vi "Cross_Moments_for_slip.vi"(0 "U":dbl[](array[numeric]) format="%.2f", 1 "W":dbl[](array[numeric]) format="%.2f", 2 "Block No":i32=1, 5 "Shift in":dbl[](array[numeric]) format="%.2f") -> (14 "Correlations Only":string[](array[string]), 19 "Shift out":dbl[](array[numeric]) format="%.2f")   [LabVIEW 2010]
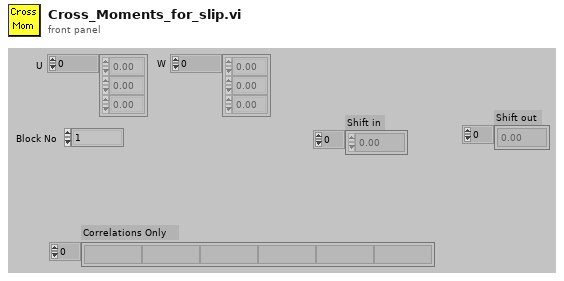
[diagram p1: front panel]
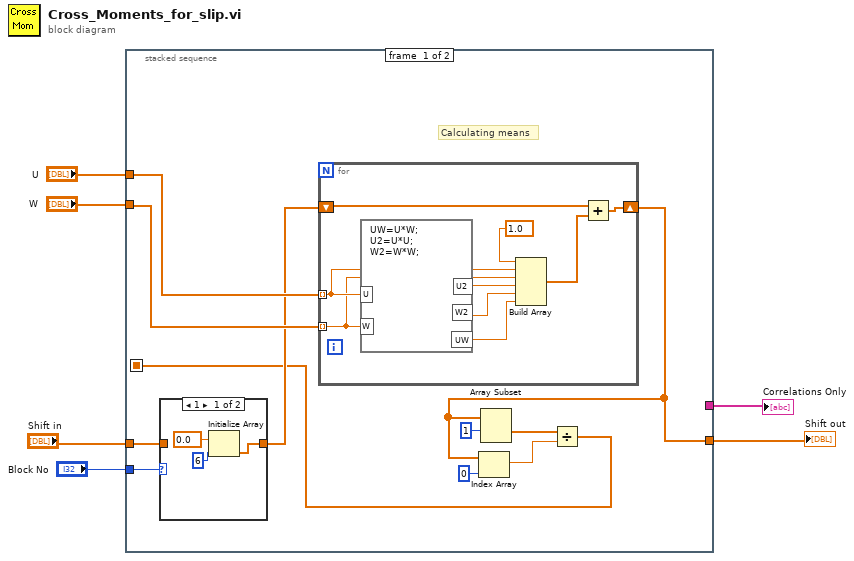
[diagram p0: block diagram]
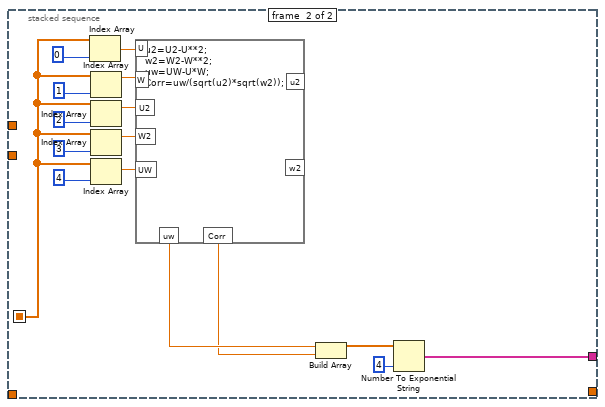
[diagram p3: hidden frame]
diagram:
  n1 = stacked-sequence {
    seq-local: [w7 _] -> [_ w41]
    tunnel: "U" -> [w17 _]
    tunnel: [w10 _] -> w5
    tunnel: "Shift in" -> [w13 _]
    tunnel: "W" -> [w16 _]
    tunnel: "Block No" -> [w15 _]
    tunnel: [_ w31] -> w1
    frame #0 {
      # "Calculating means"
      n2 = case shown="1" w15 {
        tunnel: [w18 w21] -> w14
        tunnel: w13 -> [_ w21]
        frame 1 {
          n3 = Initialize Array(0.0 ("Element Data"), 6 ("Dimension Size")) -> (w18:dbl[])
        }
        frame 2, Default {
        }
      }
      n4 = for {
        shift-right: [w26] -> w10
        shift-left: w14 -> [w25]
        tunnel: w17 -> [w24] mode=indexing
        tunnel: w16 -> [w23] mode=indexing
        n5 = formula code="UW=U*W;\nU2=U*U;\nW2=W*W;"("W"=w23, "U"=w24) -> ("UW"=w28:dbl, "U2"=w30:dbl, "W2"=w29:dbl)
        n6 = Build Array(1.0 ("Input Element"), w24, w23, w30, w29, w28) -> (w27:dbl[])
        n7 = Add(x=w25, y=w27) -> (x+y=w26:dbl[])
      }
      n8 = Index Array(array=w10, index=0 ("Index")) -> (element=w8:dbl)
      n9 = Array Subset(array=w10, index=1 ("Array Index")) -> (w9:dbl[])  [unwired: 1 in]
      n10 = Divide(x=w9, y=w8) -> (x/y=w7:dbl[])
    }
    frame #1 {
      n11 = Index Array(array=w41, index=0) -> (element=w37:dbl)
      n12 = Index Array(array=w41, index=1) -> (element=w36:dbl)
      n13 = Index Array(array=w41, index=2) -> (element=w40:dbl)
      n14 = Index Array(array=w41, index=3) -> (element=w39:dbl)
      n15 = Index Array(array=w41, index=4) -> (element=w38:dbl)
      n16 = formula code="u2=U2-U**2;\nw2=W2-W**2;\nuw=UW-U*W;\nCorr=uw/(sqrt(u2)*sqrt(w2));"("U"=w37, "W"=w36, "U2"=w40, "UW"=w38, "W2"=w39) -> ("uw"=w33:dbl, "Corr"=w32:dbl)  [unwired: 2 out]
      n17 = Build Array(w33, w32) -> (w34:dbl[])
      n18 = Number To Exponential String(number=w34, precision (6)=4) -> (E-format string=w31:string[])  [unwired: 2 out]
    }
  }
  "Shift out" <- w5
  "Correlations Only" <- w1
